vi "WT500 Set Wiring.vi"(6 "Reset Wh":bool, 7 "Crest Factor (0: 3)":u16(ring) items=["3", "6"], 8 "error in (no error)":errorcluster, 9 "Wiring (0: 1P2W, 1P2W, 1P2W)":T1=1 items=["1P2W, 1P2W, 1P2W", "1P3W, 1P2W", "3P3W, 1P2W", "1P2W, 1P3W", "1P2W, 3P3W", "3P4W", "3V3A"], 10 "Update Rate (3: 500ms)":u16(ring)=2 items=["-", "100ms", "200ms", "500ms", "1s", "2s", "5s"], 11 "VISA Refnum in":refnum<visa-resource-name>) -> (0 "error out":errorcluster, 3 "VISA Refnum out":refnum<visa-resource-name>, 5 "Instrument ID":string)   [LabVIEW 2018]
uses:
  Type Definitions/WT500 Wiring Control.ctl
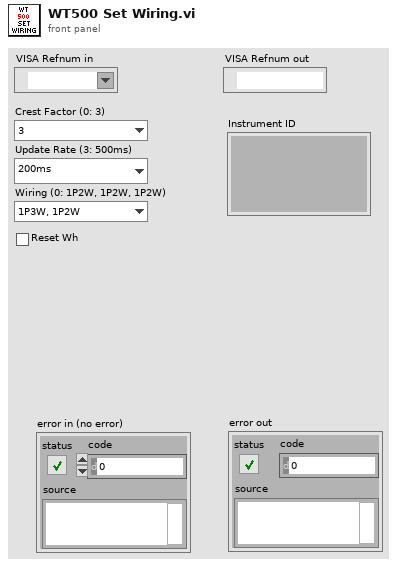
[diagram p1: front panel]
types:
  T1 = typedef "WT500 Wiring Control.ctl" = u16
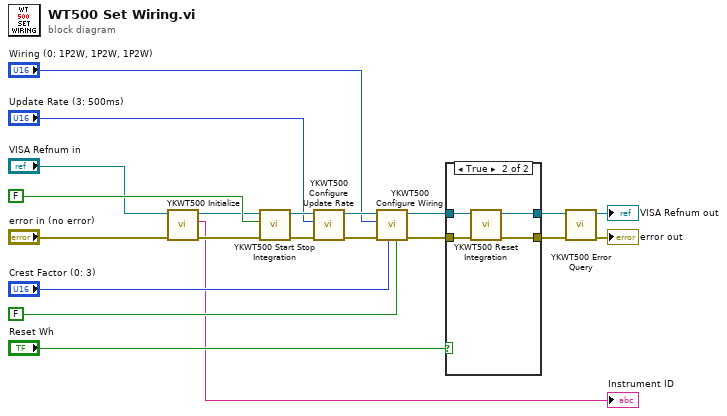
[diagram p0: block diagram]
diagram:
  n1 = call "YKWT500 Initialize.vi"("error in (no error)"="error in (no error)", "VISA resource name"="VISA Refnum in") -> ("error out"=w5:errorcluster, "Instrument ID"=→"Instrument ID":string, "VISA resource name out"=w2:refnum<visa-resource-name>)  [unwired: 7 in]
  n2 = call "YKWT500 Start Stop Integration.vi"("error in (no error)"=w5, "Start/Stop (False: Stop)"=FALSE, "VISA resource name"=w2) -> ("error out"=w17:errorcluster, "VISA resource name out"=w18:refnum<visa-resource-name>)  [unwired: 7 in]
  n3 = call "YKWT500 Configure Update Rate.vi"("error in (no error)"=w17, "Update Rate (3: 500ms)"="Update Rate (3: 500ms)", "VISA resource name"=w18) -> ("error out"=w13:errorcluster, "VISA resource name out"=w14:refnum<visa-resource-name>)  [unwired: 7 in]
  n4 = call "YKWT500 Configure Wiring.vi"("Enable Independent (False)"=FALSE, "Crest Factor (0: 3)"="Crest Factor (0: 3)", "error in (no error)"=w13, "Wiring (0: 1P2W, 1P2W, 1P2W) 2"="Wiring (0: 1P2W, 1P2W, 1P2W)", "VISA resource name"=w14) -> ("error out"=w20:errorcluster, "VISA resource name out"=w19:refnum<visa-resource-name>)  [unwired: 5 in]
  n5 = case shown="True" "Reset Wh" {
    tunnel: w20 -> [w22 w27]
    tunnel: w19 -> [w23 w26]
    tunnel: [w22 w25] -> w11
    tunnel: [w23 w24] -> w10
    frame False {
    }
    frame True {
      n6 = call "YKWT500 Reset Integration.vi"("error in (no error)"=w27, "VISA resource name"=w26) -> ("error out"=w25:errorcluster, "VISA resource name out"=w24:refnum<visa-resource-name>)  [unwired: 8 in]
    }
  }
  n7 = call "YKWT500 Error Query.vi"("error in (no error)"=w11, "VISA resource name"=w10) -> ("error out"=→"error out":errorcluster, "VISA resource name out"=→"VISA Refnum out":refnum<visa-resource-name>)  [unwired: 6 in, 2 out]
